vi "Sample Push Set Timeout.vi"(8 "error in (no error)":errorcluster, 10 "Sample Push.State Timeout":dbl, 11 "cRIO-CO2 in":refnum<class "cRIO-CO2.lvclass">) -> (0 "error out":errorcluster, 3 "cRIO-CO2 out":refnum<class "cRIO-CO2.lvclass">)   [LabVIEW 2015, in "cRIO-Carbondioxide.lvlib" / "cRIO-CO2.lvlib" / "cRIO-CO2.lvclass"]
uses:
  cRIO-CO2.lvclass
  cRIO-CO2.lvclass/cRIO-CO2.ctl
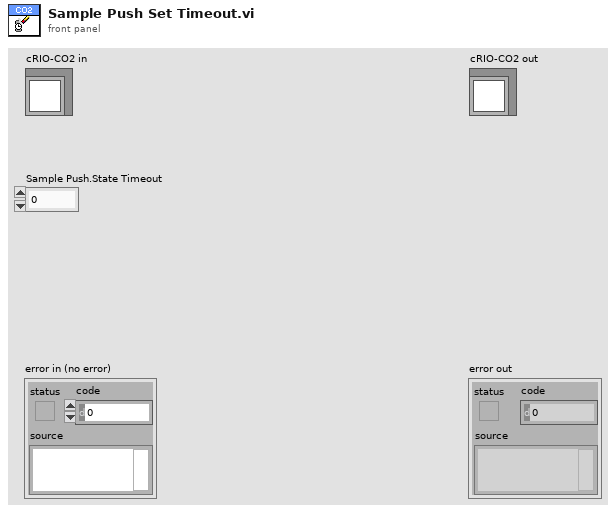
[diagram p1: front panel]
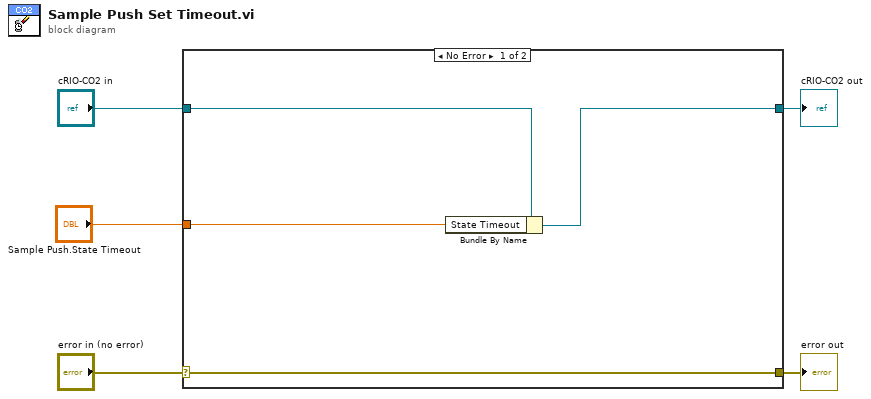
[diagram p0: block diagram]
diagram:
  n1 = case shown="No Error" "error in (no error)" {
    selector: "error in (no error)" -> [w9 w11]
    tunnel: [w9 w11] -> w4
    tunnel: [w7 w10] -> w2
    tunnel: "cRIO-CO2 in" -> [w8 w10]
    tunnel: "Sample Push.State Timeout" -> [w6 _]
    frame No Error {
      n2 = Bundle By Name(cluster=w8, "State Timeout"=w6) -> (w7:refnum<class "cRIO-CO2.lvclass">)
    }
    frame Error {
    }
  }
  "error out" <- w4
  "cRIO-CO2 out" <- w2
